vi "ackSALCommand.vi"(4 "result":string, 6 "ack":i32, 7 "CommandValue":T1, 8 "error in (no error)":errorcluster, 9 "error":i32, 10 "cmdSeqNum":i32, 11 "MiddlewareSALThisComponent in":refnum<class "MiddlewareSALThisComponent.lvclass">) -> (0 "error out":errorcluster, 3 "MiddlewareSALThisComponent out":refnum<class "MiddlewareSALThisComponent.lvclass">)   [LabVIEW 2016, in "MiddlewareSALThisComponent.lvclass"]
uses:
  MiddlewareSALThisComponent.lvclass
  Typedefs/CommandValue.ctl
  ts_sallv_sedspectrometer/DataTypes/ackcmd.ctl
  ts_sallv_sedspectrometer/SALLV_calibrationSpectrometer.lvlib
  ProgrammaticInitialization/ProgrammaticInitialization.lvclass
  Typedefs/EXATypedefs.lvlib
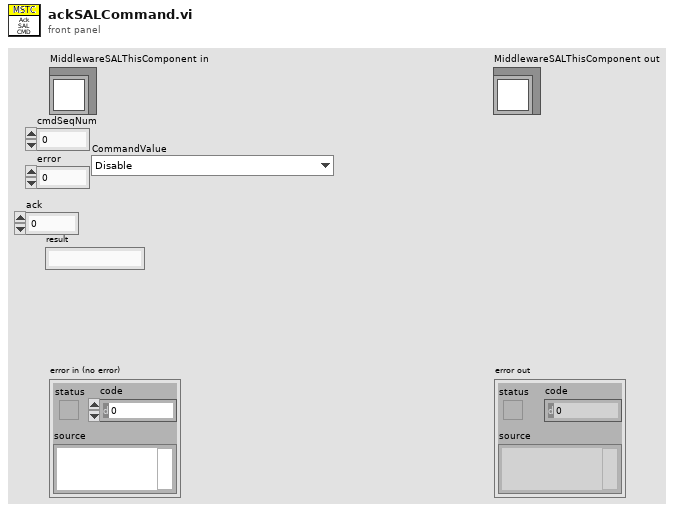
[diagram p1: front panel]
types:
  T1 = typedef "EXATypedefs.lvlib/CommandValue.ctl" = enum16{"Disable", "Enable", "Exit", "GoToStandby", "OnHeartbeat", "OnIncomingMessagingError", "OnInterrupt", "Start", "CaptureSpectImage", "SetSpectTempSetpoint", "StopImageCapture"}
  T2 = typedef "SALLV_calibrationSpectrometer.lvlib/ackcmd.ctl" = cluster{"cmdSeqNum":i32, "ack":i32, "error":i32, "result":string}
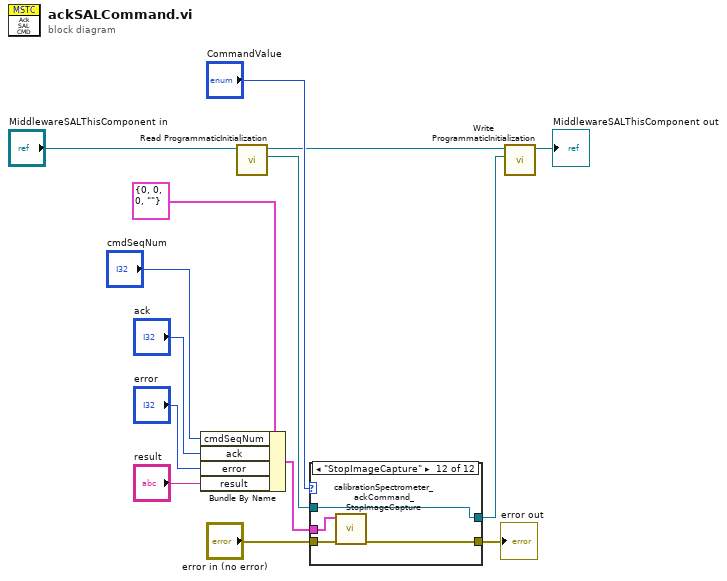
[diagram p0: block diagram]
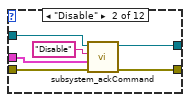
[diagram p3: hidden frame]
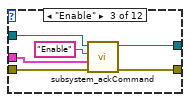
[diagram p4: hidden frame]
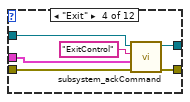
[diagram p5: hidden frame]
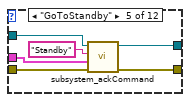
[diagram p6: hidden frame]
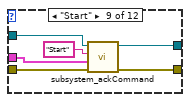
[diagram p10: hidden frame]
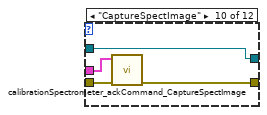
[diagram p11: hidden frame]
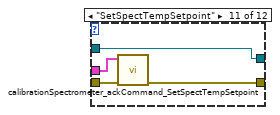
[diagram p12: hidden frame]
diagram:
  n1 = Bundle By Name(cluster=T2 {"cmdSeqNum"=0, "ack"=0, "error"=0, "result"=""} ("ackcmd_Ctl"), "cmdSeqNum"="cmdSeqNum", "ack"="ack", "error"="error", "result"="result") -> (w6:T2)
  n2 = call-dynamic "Read ProgrammaticInitialization.vi"("MiddlewareSALThisComponent in"="MiddlewareSALThisComponent in") -> ("ProgrammaticInitialization"=w4:refnum<class "ProgrammaticInitialization.lvclass">, "MiddlewareSALThisComponent out"=w2:refnum<class "MiddlewareSALThisComponent.lvclass">)  [unwired: 8 in, 1 out]
  n3 = case shown="\"StopImageCapture\"" "CommandValue" {
    tunnel: "error in (no error)" -> [w16 w21 w27 w33 w38 w42 w44 w46 w51 w55 w60 w64]
    tunnel: [w16 w22 w28 w34 w40 w42 w44 w46 w52 w54 w59 w63] -> w13
    tunnel: w6 -> [_ w20 w26 w31 w39 _ _ _ w50 w56 w57 w61]
    tunnel: w4 -> [w15 w19 w25 w32 w37 w41 w43 w45 w49 w53 w58 w62]
    tunnel: [w15 w17 w23 w29 w35 w41 w43 w45 w47 w53 w58 w62] -> w3
    frame Default {
    }
    frame "Disable" {
      n4 = call "subsystem_ackCommand.vi"("error in (no error)"=w21, "ackcmd_Ctl"=w20, "topic"="Disable", "ProgrammaticInitialization in"=w19) -> ("error out"=w22:errorcluster, "ProgrammaticInitialization out"=w17:refnum<class "ProgrammaticInitialization.lvclass">)  [unwired: 6 in]
    }
    frame "Enable" {
      n5 = call "subsystem_ackCommand.vi"("error in (no error)"=w27, "ackcmd_Ctl"=w26, "topic"="Enable", "ProgrammaticInitialization in"=w25) -> ("error out"=w28:errorcluster, "ProgrammaticInitialization out"=w23:refnum<class "ProgrammaticInitialization.lvclass">)  [unwired: 6 in]
    }
    frame "Exit" {
      n6 = call "subsystem_ackCommand.vi"("error in (no error)"=w33, "ackcmd_Ctl"=w31, "topic"="ExitControl", "ProgrammaticInitialization in"=w32) -> ("error out"=w34:errorcluster, "ProgrammaticInitialization out"=w29:refnum<class "ProgrammaticInitialization.lvclass">)  [unwired: 6 in]
    }
    frame "GoToStandby" {
      n7 = call "subsystem_ackCommand.vi"("error in (no error)"=w38, "ackcmd_Ctl"=w39, "topic"="Standby", "ProgrammaticInitialization in"=w37) -> ("error out"=w40:errorcluster, "ProgrammaticInitialization out"=w35:refnum<class "ProgrammaticInitialization.lvclass">)  [unwired: 6 in]
    }
    frame "OnHeartbeat" {
    }
    frame "OnIncomingMessagingError" {
    }
    frame "OnInterrupt" {
    }
    frame "Start" {
      n8 = call "subsystem_ackCommand.vi"("error in (no error)"=w51, "ackcmd_Ctl"=w50, "topic"="Start", "ProgrammaticInitialization in"=w49) -> ("error out"=w52:errorcluster, "ProgrammaticInitialization out"=w47:refnum<class "ProgrammaticInitialization.lvclass">)  [unwired: 6 in]
    }
    frame "CaptureSpectImage" {
      n9 = call "calibrationSpectrometer_ackCommand_CaptureSpectImage.vi"("error in (no error)"=w55, "ackcmd_Ctl"=w56) -> ("error out"=w54:errorcluster)  [unwired: 7 in, 2 out]
    }
    frame "SetSpectTempSetpoint" {
      n10 = call "calibrationSpectrometer_ackCommand_SetSpectTempSetpoint.vi"("error in (no error)"=w60, "ackcmd_Ctl"=w57) -> ("error out"=w59:errorcluster)  [unwired: 7 in, 2 out]
    }
    frame "StopImageCapture" {
      n11 = call "calibrationSpectrometer_ackCommand_StopImageCapture.vi"("error in (no error)"=w64, "ackcmd_Ctl"=w61) -> ("error out"=w63:errorcluster)  [unwired: 7 in, 2 out]
    }
  }
  "error out" <- w13
  n12 = call-dynamic "Write ProgrammaticInitialization.vi"("ProgrammaticInitialization.lvclass"=w3, "MiddlewareSALThisComponent in"=w2) -> ("MiddlewareSALThisComponent out"=→"MiddlewareSALThisComponent out":refnum<class "MiddlewareSALThisComponent.lvclass">)  [unwired: 8 in, 1 out]
